vi "Test Asic Rate Scan original con offset analogico.vi"(8 "Error IN":errorcluster, 11 "Config Test IN":T2={"Config HW"={"VISA Rigol DP832"="Rigol_DP832", "Config Rigol DP832"=[{"Channel"=0, "V Limit"=5.5, "I Limit"=0.5, "V Out"=5.0}, {"Channel"=1, "V Limit"=5.5, "I Limit"=0.8, "V Out"=5.0}, {"Channel"=2, "V Limit"=5.5, "I Limit"=0.2, "V Out"=0.0}], "CTA Test#"="CTA013 A", "FT_Handle"=0, "Espera acceso FT"=10}, "Config Test"=[{"Vasic"=2.8, "Global Reset"=FALSE, "Test Register?"=FALSE, "Test ADC?"=FALSE, "Test ADC"={"Repeats ADC"=100, "Max Desviation"=0.1}, "Limits ADC"={"Low"=[1.9, 1.3, 0.65, 0.0, 1.6, 1.4, 1.4, 0.9, 2.1, 0.85, 1.9], "High"=[2.1, 1.5, 0.85, 0.1, 1.4, 1.2, 1.2, 0.7, 1.9, 0.65, 1.7]}, "Test Max PN Min NP?"=FALSE, "Limits Max PN Min NP"={"Max P Upper"=2.177000045776367, "Min P Upper"=1.474, "Max N Upper"=1.475, "Min N Upper"=0.818, "Max P Lower"=1.888, "Min P Lower "=1.321, "Max N Lower"=1.322, "Min N Lower"=0.73}, "Test Rate Scan?"=FALSE, "Vin Rate Scan"=[], "Limits Rate Scan"={"High"=[0.15, 0.242, 0.331, 0.425, 0.512, 0.6, 0.688, 0.774, 0.847, 0.91], "Low"=[0.021, 0.11, 0.189, 0.27, 0.347, 0.421, 0.487, 0.551, 0.601, 0.635]}, "Test Rate Scan Adders?"=FALSE, "Vin Rate Adders"=[], "Limits Rate Scan adders"={"High"=[], "Low"=[]}, "Test offset analog?"=FALSE, "Lim Offset Analog"={"Max Analog"=0.05, "Min Analog"=-0.05}, "Test offset digital?"=FALSE, "Lim offset Dig"={"Max Dig"=0.05}, "Vasic real f.a."=2.8, "IBIAS"=FALSE, "VALUE IBIAS"=63}, {"Vasic"=2.8, "Global Reset"=FALSE, "Test Register?"=FALSE, "Test ADC?"=FALSE, "Test ADC"={"Repeats ADC"=100, "Max Desviation"=0.1}, "Limits ADC"={"Low"=[1.9, 1.3, 0.65, 0.0, 1.6, 1.4, 1.4, 0.9, 2.1, 0.85, 1.9], "High"=[2.1, 1.5, 0.85, 0.1, 1.4, 1.2, 1.2, 0.7, 1.9, 0.65, 1.7]}, "Test Max PN Min NP?"=FALSE, "Limits Max PN Min NP"={"Max P Upper"=2.177000045776367, "Min P Upper"=1.474, "Max N Upper"=1.475, "Min N Upper"=0.818, "Max P Lower"=1.888, "Min P Lower "=1.321, "Max N Lower"=1.322, "Min N Lower"=0.73}, "Test Rate Scan?"=FALSE, "Vin Rate Scan"=[], "Limits Rate Scan"={"High"=[0.15, 0.242, 0.331, 0.425, 0.512, 0.6, 0.688, 0.774, 0.847, 0.91], "Low"=[0.021, 0.11, 0.189, 0.27, 0.347, 0.421, 0.487, 0.551, 0.601, 0.635]}, "Test Rate Scan Adders?"=FALSE, "Vin Rate Adders"=[], "Limits Rate Scan adders"={"High"=[], "Low"=[]}, "Test offset analog?"=FALSE, "Lim Offset Analog"={"Max Analog"=0.05, "Min Analog"=-0.05}, "Test offset digital?"=FALSE, "Lim offset Dig"={"Max Dig"=0.05}, "Vasic real f.a."=2.8, "IBIAS"=FALSE, "VALUE IBIAS"=63}, {"Vasic"=2.8, "Global Reset"=FALSE, "Test Register?"=FALSE, "Test ADC?"=FALSE, "Test ADC"={"Repeats ADC"=100, "Max Desviation"=0.1}, "Limits ADC"={"Low"=[1.9, 1.3, 0.65, 0.0, 1.6, 1.4, 1.4, 0.9, 2.1, 0.85, 1.9], "High"=[2.1, 1.5, 0.85, 0.1, 1.4, 1.2, 1.2, 0.7, 1.9, 0.65, 1.7]}, "Test Max PN Min NP?"=FALSE, "Limits Max PN Min NP"={"Max P Upper"=2.177000045776367, "Min P Upper"=1.474, "Max N Upper"=1.475, "Min N Upper"=0.818, "Max P Lower"=1.888, "Min P Lower "=1.321, "Max N Lower"=1.322, "Min N Lower"=0.73}, "Test Rate Scan?"=FALSE, "Vin Rate Scan"=[], "Limits Rate Scan"={"High"=[0.15, 0.242, 0.331, 0.425, 0.512, 0.6, 0.688, 0.774, 0.847, 0.91], "Low"=[0.021, 0.11, 0.189, 0.27, 0.347, 0.421, 0.487, 0.551, 0.601, 0.635]}, "Test Rate Scan Adders?"=FALSE, "Vin Rate Adders"=[], "Limits Rate Scan adders"={"High"=[], "Low"=[]}, "Test offset analog?"=FALSE, "Lim Offset Analog"={"Max Analog"=0.05, "Min Analog"=-0.05}, "Test offset digital?"=FALSE, "Lim offset Dig"={"Max Dig"=0.05}, "Vasic real f.a."=2.8, "IBIAS"=FALSE, "VALUE IBIAS"=63}, {"Vasic"=2.8, "Global Reset"=FALSE, "Test Register?"=FALSE, "Test ADC?"=FALSE, "Test ADC"={"Repeats ADC"=100, "Max Desviation"=0.1}, "Limits ADC"={"Low"=[1.9, 1.3, 0.65, 0.0, 1.6, 1.4, 1.4, 0.9, 2.1, 0.85, 1.9], "High"=[2.1, 1.5, 0.85, 0.1, 1.4, 1.2, 1.2, 0.7, 1.9, 0.65, 1.7]}, "Test Max PN Min NP?"=FALSE, "Limits Max PN Min NP"={"Max P Upper"=2.177000045776367, "Min P Upper"=1.474, "Max N Upper"=1.475, "Min N Upper"=0.818, "Max P Lower"=1.888, "Min P Lower "=1.321, "Max N Lower"=1.322, "Min N Lower"=0.73}, "Test Rate Scan?"=FALSE, "Vin Rate Scan"=[], "Limits Rate Scan"={"High"=[0.15, 0.242, 0.331, 0.425, 0.512, 0.6, 0.688, 0.774, 0.847, 0.91], "Low"=[0.021, 0.11, 0.189, 0.27, 0.347, 0.421, 0.487, 0.551, 0.601, 0.635]}, "Test Rate Scan Adders?"=FALSE, "Vin Rate Adders"=[], "Limits Rate Scan adders"={"High"=[], "Low"=[]}, "Test offset analog?"=FALSE, "Lim Offset Analog"={"Max Analog"=0.05, "Min Analog"=-0.05}, "Test offset digital?"=FALSE, "Lim offset Dig"={"Max Dig"=0.05}, "Vasic real f.a."=2.8, "IBIAS"=FALSE, "VALUE IBIAS"=63}], "Result"=[], "Execucion Test"={"Vasic Actual"=0}, "Config VGA"={"Theoretical Voltage"=[], "Real Voltage"=[102.85, 207.14, 299.57, 404.85, 495.71, 606.85, 697.71, 801.14, 897.14, 998.85], "Pulse Width"=57344, "Frecuency Pulse"=1000000.0, "VGA Gain"=[9, 16, 24, 34, 43, 52, 61, 72, 81, 93]}, "Test Info"={"Asic"="", "Operator"="", "Place"="", "Time start"=timestamp(0 s since 1904-01-01), "Time stop"=timestamp(0 s since 1904-01-01)}, "Info machine"={"SO"="", "SO Name"="", "SO Ver"="", "SO Build"="", "CPU"="", "APP"="", "APP YEAR"="", "APP ver"="", "APP User"="", "APP Serail"="", "MAC"=[], "PC NAME"=[], "PC IP"=[], "BIOS MANU"="", "BIOS NAME"="", "BIOS SERIAL"="", "BOARD MANU"="", "BOARD NAME"="", "BOARD SERIAL"="", "Driver Version"="", "Library Version"="", "FPGA Ver"=0, "ID CTA board"=0, "LAST BOOT"="", "LABVIEW Ver"=0}} {"Config VGA"."Theoretical Voltage" format="%1.4f"; "Config VGA"."VGA Gain" format="%02x"; "Config VGA"."Frecuency Pulse" format="%0_2p"; "Config VGA"."Pulse Width" format="%04x"; "Config VGA"."Real Voltage" format="%1.5f"; "Config Test"."VALUE IBIAS" max=63 step=1; "Config Test"."Vasic real f.a." min=2.8 max=3.8 step=0.01 format="%.2g"; "Config Test"."Limits Rate Scan adders"."Low" format="%1.3f"; "Config Test"."Limits Rate Scan adders"."High" format="%1.3f"; "Config Test"."Limits ADC"."High" format="%1.4f"; "Config Test"."Limits ADC"."Low" format="%1.3f"; "Config Test"."Lim offset Dig"."Max Dig" format="%.3g"; "Config Test"."Lim Offset Analog"."Min Analog" format="%.3g"; "Config Test"."Lim Offset Analog"."Max Analog" format="%.3g"; "Config Test"."Limits Rate Scan"."Low" format="%1.4f"; "Config Test"."Limits Rate Scan"."High" format="%1.3f"; "Config Test"."Limits Max PN Min NP"."Min P Upper" format="%.3g"; "Config Test"."Limits Max PN Min NP"."Min P Lower" format="%.3g"; "Config Test"."Limits Max PN Min NP"."Max N Lower" format="%.3g"; "Config Test"."Limits Max PN Min NP"."Max N Upper" format="%.3g"; "Config Test"."Limits Max PN Min NP"."Min N Lower" format="%.3g"; "Config Test"."Limits Max PN Min NP"."Min N Upper" format="%.3g"; "Config Test"."Limits Max PN Min NP"."Max P Upper" format="%.3g"; "Config Test"."Limits Max PN Min NP"."Max P Lower" format="%.3g"; "Config Test"."Vasic" min=2.8 max=3.8 step=0.01 format="%.2g"; "Config HW"."Config Rigol DP832"."Channel" items=["+30V Channel 1", "+30V Channel 2", "+5V Channel 3"]; "Config HW"."Config Rigol DP832"."V Limit" format="%.1g"; "Config HW"."Config Rigol DP832"."I Limit" format="%.1g"; "Config HW"."Config Rigol DP832"."V Out" format="%.1g"; "Result"."Test Registros"."Read W/R" format="%04x"; "Result"."Test Registros"."Pattern W/R" format="%04x"; "Result"."Test Registros"."Read Default" format="%04x"; "Result"."Test Registros"."Pattern Default" format="%04x"}) -> (0 "Error OUT":errorcluster, 2 "Rate scan all ok":bool, 3 "Config Test OUT":T2={"Config HW"={"VISA Rigol DP832"="Rigol_DP832", "Config Rigol DP832"=[{"Channel"=0, "V Limit"=5.5, "I Limit"=0.5, "V Out"=5.0}, {"Channel"=1, "V Limit"=5.5, "I Limit"=0.8, "V Out"=5.0}, {"Channel"=2, "V Limit"=5.5, "I Limit"=0.2, "V Out"=0.0}], "CTA Test#"="CTA013 A", "FT_Handle"=0, "Espera acceso FT"=10}, "Config Test"=[{"Vasic"=2.8, "Global Reset"=FALSE, "Test Register?"=FALSE, "Test ADC?"=FALSE, "Test ADC"={"Repeats ADC"=100, "Max Desviation"=0.1}, "Limits ADC"={"Low"=[1.9, 1.3, 0.65, 0.0, 1.6, 1.4, 1.4, 0.9, 2.1, 0.85, 1.9], "High"=[2.1, 1.5, 0.85, 0.1, 1.4, 1.2, 1.2, 0.7, 1.9, 0.65, 1.7]}, "Test Max PN Min NP?"=FALSE, "Limits Max PN Min NP"={"Max P Upper"=2.177000045776367, "Min P Upper"=1.474, "Max N Upper"=1.475, "Min N Upper"=0.818, "Max P Lower"=1.888, "Min P Lower "=1.321, "Max N Lower"=1.322, "Min N Lower"=0.73}, "Test Rate Scan?"=FALSE, "Vin Rate Scan"=[], "Limits Rate Scan"={"High"=[0.15, 0.242, 0.331, 0.425, 0.512, 0.6, 0.688, 0.774, 0.847, 0.91], "Low"=[0.021, 0.11, 0.189, 0.27, 0.347, 0.421, 0.487, 0.551, 0.601, 0.635]}, "Test Rate Scan Adders?"=FALSE, "Vin Rate Adders"=[], "Limits Rate Scan adders"={"High"=[], "Low"=[]}, "Test offset analog?"=FALSE, "Lim Offset Analog"={"Max Analog"=0.05, "Min Analog"=-0.05}, "Test offset digital?"=FALSE, "Lim offset Dig"={"Max Dig"=0.05}, "Vasic real f.a."=2.8, "IBIAS"=FALSE, "VALUE IBIAS"=63}, {"Vasic"=2.8, "Global Reset"=FALSE, "Test Register?"=FALSE, "Test ADC?"=FALSE, "Test ADC"={"Repeats ADC"=100, "Max Desviation"=0.1}, "Limits ADC"={"Low"=[1.9, 1.3, 0.65, 0.0, 1.6, 1.4, 1.4, 0.9, 2.1, 0.85, 1.9], "High"=[2.1, 1.5, 0.85, 0.1, 1.4, 1.2, 1.2, 0.7, 1.9, 0.65, 1.7]}, "Test Max PN Min NP?"=FALSE, "Limits Max PN Min NP"={"Max P Upper"=2.177000045776367, "Min P Upper"=1.474, "Max N Upper"=1.475, "Min N Upper"=0.818, "Max P Lower"=1.888, "Min P Lower "=1.321, "Max N Lower"=1.322, "Min N Lower"=0.73}, "Test Rate Scan?"=FALSE, "Vin Rate Scan"=[], "Limits Rate Scan"={"High"=[0.15, 0.242, 0.331, 0.425, 0.512, 0.6, 0.688, 0.774, 0.847, 0.91], "Low"=[0.021, 0.11, 0.189, 0.27, 0.347, 0.421, 0.487, 0.551, 0.601, 0.635]}, "Test Rate Scan Adders?"=FALSE, "Vin Rate Adders"=[], "Limits Rate Scan adders"={"High"=[], "Low"=[]}, "Test offset analog?"=FALSE, "Lim Offset Analog"={"Max Analog"=0.05, "Min Analog"=-0.05}, "Test offset digital?"=FALSE, "Lim offset Dig"={"Max Dig"=0.05}, "Vasic real f.a."=2.8, "IBIAS"=FALSE, "VALUE IBIAS"=63}, {"Vasic"=2.8, "Global Reset"=FALSE, "Test Register?"=FALSE, "Test ADC?"=FALSE, "Test ADC"={"Repeats ADC"=100, "Max Desviation"=0.1}, "Limits ADC"={"Low"=[1.9, 1.3, 0.65, 0.0, 1.6, 1.4, 1.4, 0.9, 2.1, 0.85, 1.9], "High"=[2.1, 1.5, 0.85, 0.1, 1.4, 1.2, 1.2, 0.7, 1.9, 0.65, 1.7]}, "Test Max PN Min NP?"=FALSE, "Limits Max PN Min NP"={"Max P Upper"=2.177000045776367, "Min P Upper"=1.474, "Max N Upper"=1.475, "Min N Upper"=0.818, "Max P Lower"=1.888, "Min P Lower "=1.321, "Max N Lower"=1.322, "Min N Lower"=0.73}, "Test Rate Scan?"=FALSE, "Vin Rate Scan"=[], "Limits Rate Scan"={"High"=[0.15, 0.242, 0.331, 0.425, 0.512, 0.6, 0.688, 0.774, 0.847, 0.91], "Low"=[0.021, 0.11, 0.189, 0.27, 0.347, 0.421, 0.487, 0.551, 0.601, 0.635]}, "Test Rate Scan Adders?"=FALSE, "Vin Rate Adders"=[], "Limits Rate Scan adders"={"High"=[], "Low"=[]}, "Test offset analog?"=FALSE, "Lim Offset Analog"={"Max Analog"=0.05, "Min Analog"=-0.05}, "Test offset digital?"=FALSE, "Lim offset Dig"={"Max Dig"=0.05}, "Vasic real f.a."=2.8, "IBIAS"=FALSE, "VALUE IBIAS"=63}, {"Vasic"=2.8, "Global Reset"=FALSE, "Test Register?"=FALSE, "Test ADC?"=FALSE, "Test ADC"={"Repeats ADC"=100, "Max Desviation"=0.1}, "Limits ADC"={"Low"=[1.9, 1.3, 0.65, 0.0, 1.6, 1.4, 1.4, 0.9, 2.1, 0.85, 1.9], "High"=[2.1, 1.5, 0.85, 0.1, 1.4, 1.2, 1.2, 0.7, 1.9, 0.65, 1.7]}, "Test Max PN Min NP?"=FALSE, "Limits Max PN Min NP"={"Max P Upper"=2.177000045776367, "Min P Upper"=1.474, "Max N Upper"=1.475, "Min N Upper"=0.818, "Max P Lower"=1.888, "Min P Lower "=1.321, "Max N Lower"=1.322, "Min N Lower"=0.73}, "Test Rate Scan?"=FALSE, "Vin Rate Scan"=[], "Limits Rate Scan"={"High"=[0.15, 0.242, 0.331, 0.425, 0.512, 0.6, 0.688, 0.774, 0.847, 0.91], "Low"=[0.021, 0.11, 0.189, 0.27, 0.347, 0.421, 0.487, 0.551, 0.601, 0.635]}, "Test Rate Scan Adders?"=FALSE, "Vin Rate Adders"=[], "Limits Rate Scan adders"={"High"=[], "Low"=[]}, "Test offset analog?"=FALSE, "Lim Offset Analog"={"Max Analog"=0.05, "Min Analog"=-0.05}, "Test offset digital?"=FALSE, "Lim offset Dig"={"Max Dig"=0.05}, "Vasic real f.a."=2.8, "IBIAS"=FALSE, "VALUE IBIAS"=63}], "Result"=[], "Execucion Test"={"Vasic Actual"=0}, "Config VGA"={"Theoretical Voltage"=[], "Real Voltage"=[102.85, 207.14, 299.57, 404.85, 495.71, 606.85, 697.71, 801.14, 897.14, 998.85], "Pulse Width"=57344, "Frecuency Pulse"=1000000.0, "VGA Gain"=[9, 16, 24, 34, 43, 52, 61, 72, 81, 93]}, "Test Info"={"Asic"="", "Operator"="", "Place"="", "Time start"=timestamp(0 s since 1904-01-01), "Time stop"=timestamp(0 s since 1904-01-01)}, "Info machine"={"SO"="", "SO Name"="", "SO Ver"="", "SO Build"="", "CPU"="", "APP"="", "APP YEAR"="", "APP ver"="", "APP User"="", "APP Serail"="", "MAC"=[], "PC NAME"=[], "PC IP"=[], "BIOS MANU"="", "BIOS NAME"="", "BIOS SERIAL"="", "BOARD MANU"="", "BOARD NAME"="", "BOARD SERIAL"="", "Driver Version"="", "Library Version"="", "FPGA Ver"=0, "ID CTA board"=0, "LAST BOOT"="", "LABVIEW Ver"=0}} {"Config VGA"."Theoretical Voltage" format="%1.4f"; "Config VGA"."VGA Gain" format="%02x"; "Config VGA"."Frecuency Pulse" format="%0_2p"; "Config VGA"."Pulse Width" format="%04x"; "Config VGA"."Real Voltage" format="%1.5f"; "Config Test"."VALUE IBIAS" max=63 step=1; "Config Test"."Vasic real f.a." min=2.8 max=3.8 step=0.01 format="%.2g"; "Config Test"."Limits Rate Scan adders"."Low" format="%1.3f"; "Config Test"."Limits Rate Scan adders"."High" format="%1.3f"; "Config Test"."Limits ADC"."High" format="%1.4f"; "Config Test"."Limits ADC"."Low" format="%1.3f"; "Config Test"."Lim offset Dig"."Max Dig" format="%.3g"; "Config Test"."Lim Offset Analog"."Min Analog" format="%.3g"; "Config Test"."Lim Offset Analog"."Max Analog" format="%.3g"; "Config Test"."Limits Rate Scan"."Low" format="%1.4f"; "Config Test"."Limits Rate Scan"."High" format="%1.3f"; "Config Test"."Limits Max PN Min NP"."Min P Upper" format="%.3g"; "Config Test"."Limits Max PN Min NP"."Min P Lower" format="%.3g"; "Config Test"."Limits Max PN Min NP"."Max N Lower" format="%.3g"; "Config Test"."Limits Max PN Min NP"."Max N Upper" format="%.3g"; "Config Test"."Limits Max PN Min NP"."Min N Lower" format="%.3g"; "Config Test"."Limits Max PN Min NP"."Min N Upper" format="%.3g"; "Config Test"."Limits Max PN Min NP"."Max P Upper" format="%.3g"; "Config Test"."Limits Max PN Min NP"."Max P Lower" format="%.3g"; "Config Test"."Vasic" min=2.8 max=3.8 step=0.01 format="%.2g"; "Config HW"."Config Rigol DP832"."Channel" items=["+30V Channel 1", "+30V Channel 2", "+5V Channel 3"]; "Config HW"."Config Rigol DP832"."V Limit" format="%.1g"; "Config HW"."Config Rigol DP832"."I Limit" format="%.1g"; "Config HW"."Config Rigol DP832"."V Out" format="%.1g"; "Result"."Test Registros"."Read W/R" format="%04x"; "Result"."Test Registros"."Pattern W/R" format="%04x"; "Result"."Test Registros"."Read Default" format="%04x"; "Result"."Test Registros"."Pattern Default" format="%04x"})   [LabVIEW 2009]
uses:
  Test.ctl
  TEST.TEST CONFIG HW.ctl
  Rigol DP832/DP832_Control Channels.ctl
  TEST.TEST CONFIG TEST MATRIZ.ctl
  TEST.TEST CONFIG TEST.ctl
  TEST.TEST RESULT.ctl
  test_result fvasic.ctl
  TEST.TEST EXECUTION TEST.ctl
  TEST.TEST CONFIG VGA.ctl
  TEST.TEST TEST INFO.ctl
  TEST.TEST INFO PC.ctl
  Global.Salir Ya.vi
panel:
  out "subarray":dbl[][](array[numeric])
  in  "DAC\nTH0,TH1,TH2":u16
  in  "Tab Control":enum32{"Page 1", "Page 2"}(tab)
  out "%":u8 format="%02d%%"
  out "B":u8(slide) scale=0.0..100.0
  out "Indicador":string
  out "Comparation LLTH":bool[][][](array[boolean])
  out "Comparation HLTH":bool[][][](array[boolean])
  out "Reference":T1
  out "DAC TH3,TH4,TH5":u16
  out "LLTHx":dbl
  out "DAC TH0,TH1,TH2":u16
  out "HLTHx":dbl
  out "Volt LLTH (salida B)":dbl[][][](array[numeric])
  out "Volt HLTH (salida A)":dbl[][][](array[numeric])
  out "DAC TH3,TH4,TH5":u16[][][](array[numeric])
  out "DAC TH0,TH1,TH2":u16[][][](array[numeric])
  # "Vin Asic"
  # "Canal"
  # "Sumador"
  # "Test ASIC. Rate Scan"
  # "Modo 2\nModo 3\nModo 4\nModo 2\nModo 3\nModo 4"
  # "Modo 2\nModo 3\nModo 4\nModo 2\nModo 3\nModo 4"
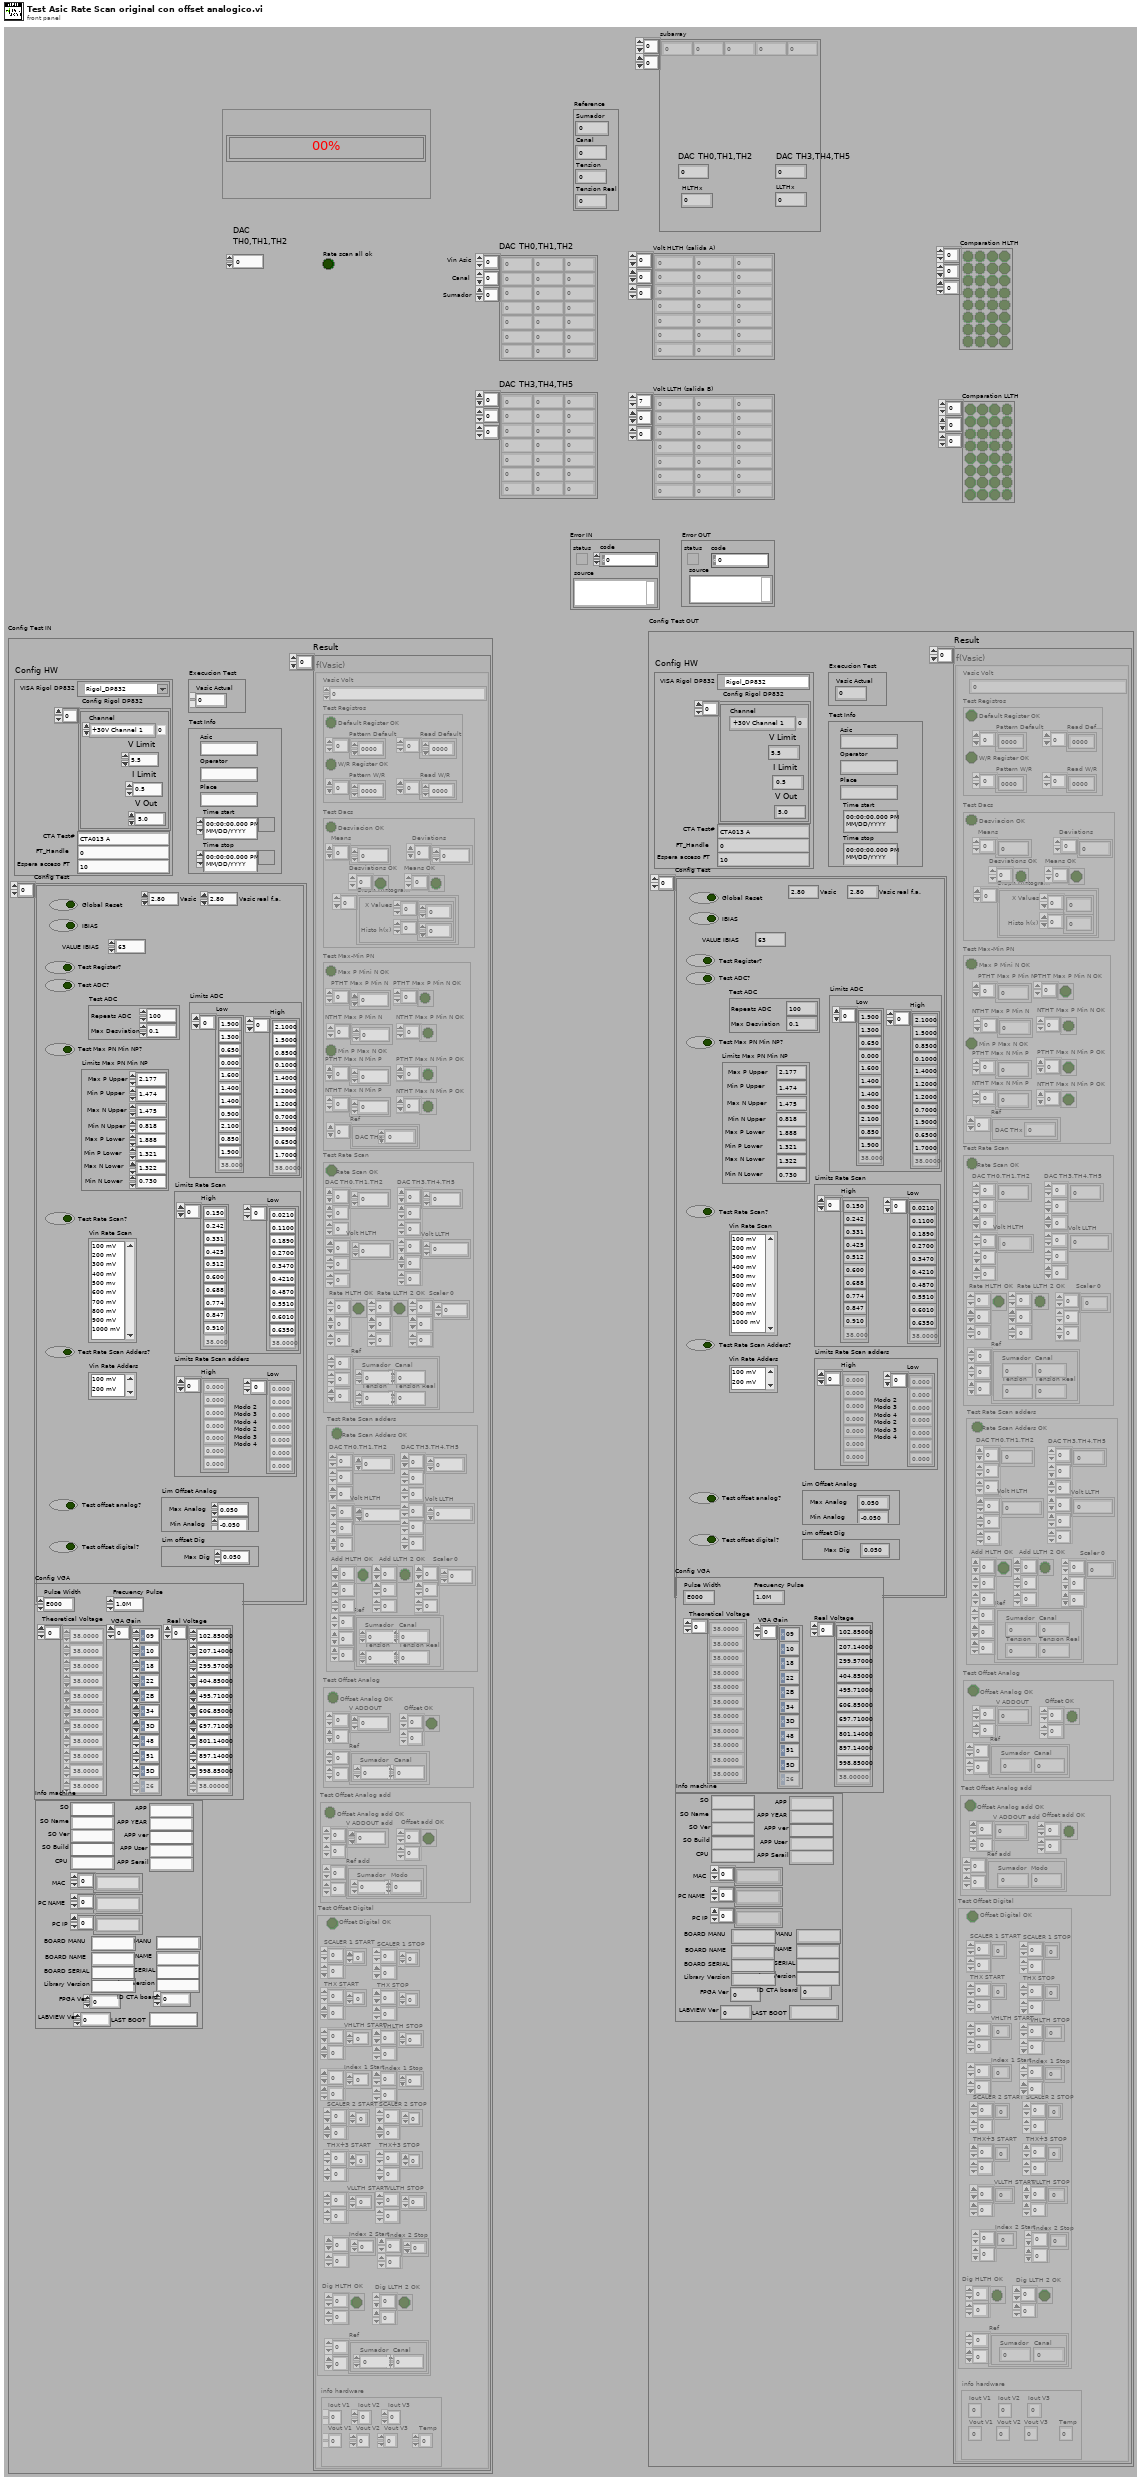
[diagram p1: front panel]
types:
  T1 = cluster{"Sumador":u8, "Canal":u8, "Tension":u8, "Tension Real":dbl}
  T2 = typedef "Test.ctl" = cluster{"Config HW":T3, "Config Test":T5, "Result":T7, "Execucion Test":T9, "Config VGA":T10, "Test Info":T11, "Info machine":T12}
  T3 = typedef "TEST.TEST CONFIG HW.ctl" = cluster{"VISA Rigol DP832":refnum<visa-resource-name>, "Config Rigol DP832":cluster{"Channel":T4, "V Limit":dbl, "I Limit":dbl, "V Out":dbl}[], "CTA Test#":string, "FT_Handle":u32, "Espera acceso FT":u32}
  T4 = typedef "DP832_Control Channels.ctl" = i32
  T5 = typedef "TEST.TEST CONFIG TEST MATRIZ.ctl" = T6[]
  T6 = typedef "TEST.TEST CONFIG TEST.ctl" = cluster{"Vasic":dbl, "Global Reset":bool, "Test Register?":bool, "Test ADC?":bool, "Test ADC":cluster{"Repeats ADC":i32, "Max Desviation":dbl}, "Limits ADC":cluster{"Low":dbl[], "High":dbl[]}, "Test Max PN Min NP?":bool, "Limits Max PN Min NP":cluster{"Max P Upper":dbl, "Min P Upper":dbl, "Max N Upper":dbl, "Min N Upper":dbl, "Max P Lower":dbl, "Min P Lower ":dbl, "Max N Lower":dbl, "Min N Lower":dbl}, "Test Rate Scan?":bool, "Vin Rate Scan":i32[], "Limits Rate Scan":cluster{"High":dbl[], "Low":dbl[]}, "Test Rate Scan Adders?":bool, "Vin Rate Adders":i32[], "Limits Rate Scan adders":cluster{"High":dbl[], "Low":dbl[]}, "Test offset analog?":bool, "Lim Offset Analog":cluster{"Max Analog":dbl, "Min Analog":dbl}, "Test offset digital?":bool, "Lim offset Dig":cluster{"Max Dig":dbl}, "Vasic real f.a.":dbl, "IBIAS":bool, "VALUE IBIAS":u8}
  T7 = typedef "TEST.TEST RESULT.ctl" = T8[]
  T8 = typedef "test_result fvasic.ctl" = cluster{"Vasic Volt":i32, "Test Registros":cluster{"Default Register OK":bool, "Pattern Default":u16[], "Read Default":u16[], "W/R Register OK":bool, "Pattern W/R":u16[], "Read W/R":u16[]}, "Test Dacs":cluster{"Desviacion OK":bool, "Means":dbl[], "Deviations":dbl[], "Desviations OK":bool[], "Means OK":bool[], "Graph Histogram":cluster{"X Values":dbl[], "Histo h(x)":i32[]}[]}, "Test Max-Min PN":cluster{"Max P Mini N OK":bool, "PTHT Max P Min N":dbl[], "PTHT Max P Min N OK":bool[], "NTHT Max P Min N":dbl[], "NTHT Max P Min N OK":bool[], "Min P Max N OK":bool, "PTHT Max N Min P":dbl[], "PTHT Max N Min P OK":bool[], "NTHT Max N Min P":dbl[], "NTHT Max N Min P OK":bool[], "Ref":cluster{"DAC THx":u8}[]}, "Test Rate Scan":cluster{"Rate Scan OK":bool, "DAC TH0,TH1,TH2":u16[][][], "Volt HLTH":dbl[][][], "Rate HLTH OK":bool[][][], "DAC TH3,TH4,TH5":u16[][][], "Volt LLTH":dbl[][][], "Rate LLTH 2 OK":bool[][][], "Scaler 0":u16[][][], "Ref":cluster{"Sumador":u8, "Canal":u8, "Tension":u8, "Tension Real":dbl}[][][]}, "Test Rate Scan adders":cluster{"Rate Scan Adders OK":bool, "DAC TH0,TH1,TH2":u16[][][], "Volt HLTH":dbl[][][], "Add HLTH OK":bool[][][], "DAC TH3,TH4,TH5":u16[][][], "Volt LLTH":dbl[][][], "Add LLTH 2 OK":bool[][][], "Scaler 0":u16[][][], "Ref":cluster{"Sumador":u8, "Canal":u8, "Tension":u8, "Tension Real":dbl}[][][]}, "Test Offset Analog":cluster{"Offset Analog OK":bool, "V ADDOUT":dbl[][], "Offset OK":bool[][], "Ref":cluster{"Sumador":u8, "Canal":u8}[][]}, "Test Offset Digital":cluster{"Offset Digital OK":bool, "SCALER 1 START":u16[][], "SCALER 1 STOP":u16[][], "THX START":u16[][], "THX STOP":u16[][], "VHLTH START":dbl[][], "VHLTH STOP":dbl[][], "Index 1 Start":i32[][], "index 1 Stop":i32[][], "SCALER 2 START":u16[][], "SCALER 2 STOP":u16[][], "THX+3 START":u16[][], "THX+3 STOP":u16[][], "VLLTH START":dbl[][], "VLLTH STOP":dbl[][], "Index 2 Start":i32[][], "index 2 Stop":i32[][], "Dig HLTH OK":bool[][], "Dig LLTH 2 OK":bool[][], "Ref":cluster{"Sumador":u8, "Canal":u8}[][]}, "info hardware":cluster{"Iout V1":dbl, "Iout V2":dbl, "Iout V3":dbl, "Vout V1":dbl, "Vout V2":dbl, "Vout V3":dbl, "Temp":dbl}, "Test Offset Analog add":cluster{"Offset Analog add OK":bool, "V ADDOUT add":dbl[][], "Offset add OK":bool[][], "Ref add":cluster{"Sumador":u8, "Modo":u8}[][]}}
  T9 = typedef "TEST.TEST EXECUTION TEST.ctl" = cluster{"Vasic Actual":i32}
  T10 = typedef "TEST.TEST CONFIG VGA.ctl" = cluster{"Theoretical Voltage":dbl[], "Real Voltage":dbl[], "Pulse Width":u16, "Frecuency Pulse":dbl, "VGA Gain":u8[]}
  T11 = typedef "TEST.TEST TEST INFO.ctl" = cluster{"Asic":string, "Operator":string, "Place":string, "Time start":timestamp, "Time stop":timestamp}
  T12 = typedef "TEST.TEST INFO PC.ctl" = cluster{"SO":string, "SO Name":string, "SO Ver":string, "SO Build":string, "CPU":string, "APP":string, "APP YEAR":string, "APP ver":string, "APP User":string, "APP Serail":string, "MAC":string[], "PC NAME":string[], "PC IP":string[], "BIOS MANU":string, "BIOS NAME":string, "BIOS SERIAL":string, "BOARD MANU":string, "BOARD NAME":string, "BOARD SERIAL":string, "Driver Version":string, "Library Version":string, "FPGA Ver":u8, "ID CTA board":u64, "LAST BOOT":string, "LABVIEW Ver":u32}
  T13 = enum16{"Always On", "Always Off", "Off While Running"}
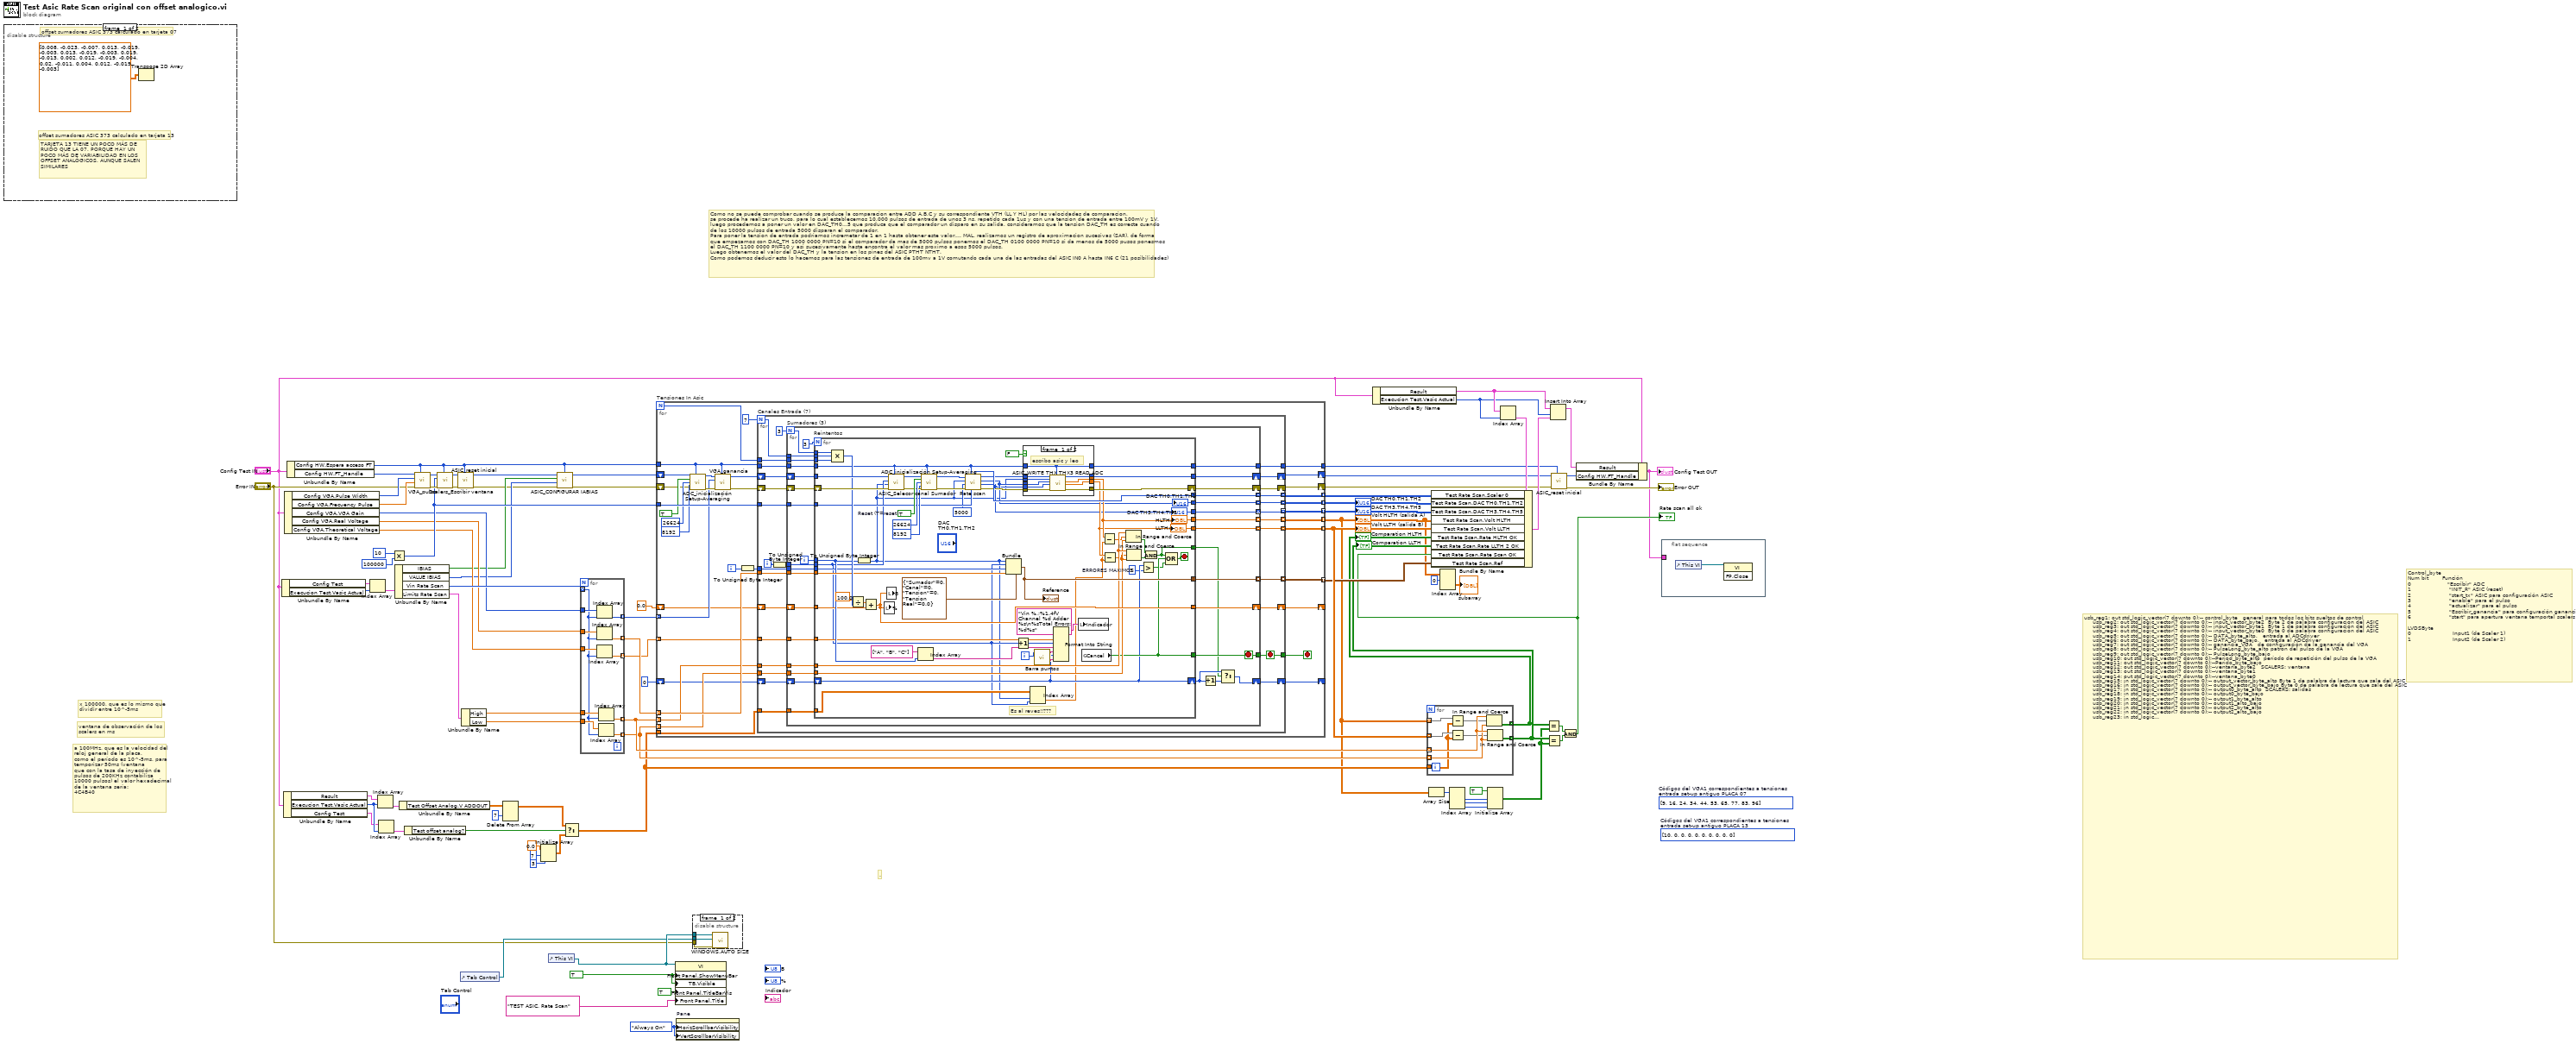
[diagram p0: block diagram]
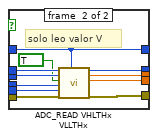
[diagram p4: hidden frame]
diagram:
  w1 = T13."Always On" ("Horizontal Scrollbar Visibility")
  w41 = TRUE ("Front Panel Window:Show Menu Bar")
  (unwired) u8[] [10, 0, 0, 0, 0, 0, 0, 0, 0, 0]  # Códigos del VGA1 correspondientes a tensiones entrada set-up antiguo PLACA 13
  (unwired) u8[] [9, 16, 24, 34, 44, 53, 65, 77, 83, 96]  # Códigos del VGA1 correspondientes a tensiones entrada set-up antiguo PLACA 07
  # "."
  # "Como no se puede comprobar cuando se produce la comparacion entre ADD A,B,C y su correspondiente VTH (LL Y HL) por las velocidades de comparacion,\nse procede ha realizar un truco, para lo cual establecemos 10.000 pulsos de entrada de unos 3 ns, repetido cada 1us y con una tension de entrada entre 100mV y 1V,\nluego procedemos a poner un valor en DAC_TH0...5 que produca que el comparador un disparo en su salida, consideramos que la tension DAC_TH es correcta cuando\nde los 10000 pulsos de entrada 5000 disparan el comparador.\nPara poner la tension de entrada podriamos incremetar de 1 en 1 hasta obtener este valor.... MAL. realizamos un registro de aproximacion sucesivas (SAR), de forma\nque empezamos con DAC_TH 1000 0000 PN=10 si el comparador da mas de 5000 pulsos ponemos el DAC_TH 0100 0000 PN=10 si da menos de 5000 pusos ponesmos\nel DAC_TH 1100 0000 PN=10 y asi sucesivamente hasta encontra el valor mas proximo a esos 5000 pulsos. \nLuego obtenemos el valor del DAC_TH y la tension en los pines del ASIC PTHT NTHT.\nComo podemos deducir esto lo hacemos para las tensiones de entrada de 100mv a 1V comutando cada una de las entradas del ASIC IN0 A hasta IN6 C (21 posibilidades)"
  # "Control_byte\nNum bit        Función\n0                     \"Escribir\" ADC\n1                      \"INIT_R\" ASIC (reset)\n2                      \"start_tx\" ASIC para configuración ASIC\n3                      \"enable\" para el pulso\n4                      \"actualizar\" para el pulso\n5                      \"Escribir_ganancia\" para configuración ganancia\n6                      \"start\" para apertura ventana temportal scalers\n\nLVDSByte\n0                        Input1 (de Scaler 1)\n1                        Input2 (de Scaler 2)"
  # "usb_reg1: out std_logic_vector(7 downto 0);-- control_byte\t\t\tgeneral para todos los bits sueltos de control\n\t\t\t  usb_reg2: out std_logic_vector(7 downto 0);-- input_vector_byte2 \tByte 2 de palabra configuración del ASIC\n\t\t\t  usb_reg3: out std_logic_vector(7 downto 0);-- input_vector_byte1 \tByte 1 de palabra configuración del ASIC\n\t\t\t  usb_reg4: out std_logic_vector(7 downto 0);-- input_vector_byte0 \tByte 0 de palabra configuración del ASIC\n\t\t\t  usb_reg5: out std_logic_vector(7 downto 0);-- DATA_byte_alto, \t\tentrada al ADCdriver\n\t\t\t  usb_reg6: out std_logic_vector(7 downto 0);-- DATA_byte_bajo, \t\tentrada al ADCdriver\n\t\t\t  usb_reg7: out std_logic_vector(7 downto 0);-- ganancia_VGA\t\t\tde configuración de la ganancia del VGA\n\t\t\t  usb_reg8: out std_logic_vector(7 downto 0);-- PulseLong_byte_alto\tpatrón del pulso de la VGA\n\t\t\t  usb_reg9: out std_logic_vector(7 downto 0);-- PulseLong_byte_bajo\n\t\t\t  usb_reg10: out std_logic_vector(7 downto 0);--Period_byte_alto\t\tperíodo de repetición del pulso de la VGA\n\t\t\t  usb_reg11: out std_logic_vector(7 downto 0);--Perido_byte_bajo\n\t\t\t  usb_reg12: out std_logic_vector(7 downto 0);--ventana_byte2\t\t\tSCALERS: ventana\n\t\t\t  usb_reg13: out std_logic_vector(7 downto 0);--ventana_byte1\t\n\t\t\t  usb_reg14: out std_logic_vector(7 downto 0);--ventana_byte0\n\t\t\t  usb_reg15: in std_logic_vector(7 downto 0);-- output_vector_byte_alto\tByte 1 de palabra de lectura que sale del ASIC\n\t\t\t  usb_reg16: in std_logic_vector(7 downto 0);-- output_vector_byte_bajo\tByte 0 de palabra de lectura que sale del ASIC\n\t\t\t  usb_reg17: in std_logic_vector(7 downto 0);-- output0_byte_alto\t\tSCALERS: salidas\n\t\t\t  usb_reg18: in std_logic_vector(7 downto 0);-- output0_byte_bajo\n\t\t\t  usb_reg19: in std_logic_vector(7 downto 0);-- output1_byte_alto\n\t\t\t  usb_reg20: in std_logic_vector(7 downto 0);-- output1_alto_bajo \n\t\t\t  usb_reg21: in std_logic_vector(7 downto 0);-- output2_byte_alto \n\t\t\t  usb_reg22: in std_logic_vector(7 downto 0);-- output2_alto_bajo \n\t\t\t  usb_reg23: in std_logic_vector(7 downto 0);-- para el canal_0 del ADCdriver\n\t\t\t  usb_reg24: in std_logic_vector(7 downto 0);\n\t\t\t  usb_reg25: in std_logic_vector(7 downto 0);-- para el canal_1 del ADCdriver\n\t\t\t  usb_reg26: in std_logic_vector(7 downto 0);\n\t\t\t  usb_reg27: in std_logic_vector(7 downto 0);-- para el canal_2 del ADCdriver\n\t\t\t  usb_reg28: in std_logic_vector(7 downto 0);\n\t\t\t  usb_reg29: in std_logic_vector(7 downto 0);-- para el canal_3 del ADCdriver\n\t\t\t  usb_reg30: in std_logic_vector(7 downto 0);\n\t\t\t  usb_reg31: in std_logic_vector(7 downto 0);-- para el canal_4 del ADCdriver\n\t\t\t  usb_reg32: in std_logic_vector(7 downto 0);\n\t\t\t  usb_reg33: in std_logic_vector(7 downto 0);-- para el canal_5 del ADCdriver\n\t\t\t  usb_reg34: in std_logic_vector(7 downto 0);\n\t\t\t  usb_reg35: in std_logic_vector(7 downto 0);-- para el canal_6 del ADCdriver\n\t\t\t  usb_reg36: in std_logic_vector(7 downto 0);\n\t\t\t  usb_reg37: in std_logic_vector(7 downto 0);-- para el canal_7 del ADCdriver\n\t\t\t  usb_reg38: in std_logic_vector(7 downto 0);\n\t\t\t  usb_reg39: in std_logic_vector(7 downto 0);-- para el canal_8 del ADCdriver\n\t\t\t  usb_reg40: in std_logic_vector(7 downto 0);\n\t\t\t  usb_reg41: in std_logic_vector(7 downto 0);-- para el canal_9 del ADCdriver\n\t\t\t  usb_reg42: in std_logic_vector(7 downto 0);\n\t\t\t  usb_reg43: in std_logic_vector(7 downto 0);-- para el canal_10 del ADCdriver\n\t\t\t  usb_reg44: in std_logic_vector(7 downto 0)--;  \n\n     usb_reg55 => LVDSByte"
  # "x 100000, que es lo mismo que dividir entre 10^-5ms"
  # "ventana de observación de los scalers en ms"
  # "a 100MHz, que es la velocidad del reloj general de la placa,\ncomo el período es 10^-5ms, para temporizar 50ms (ventana \nque con la tasa de inyección de pulsos de 200KHz contabiliza \n10000 pulsos) el valor hexadecimal de la ventana sería:\n4C4B40"
  n1 = disable-structure shown="Enabled" {
    frame #0 {
      # "TARJETA 13 TIENE UN POCO MÁS DE \nRUIDO QUE LA 07, PORQUE HAY UN\nPOCO MÁS DE VARIABILIDAD EN LOS \nOFFSET ANALÓGICOS, AUNQUE SALEN\nSIMILARES"
      # "offset sumadores ASIC 373 calculado en tarjeta 13"
      # "offset sumadores ASIC 373 calculado en tarjeta 07"
      n2 = Transpose 2D Array(2D array=dbl[][] [[0.008, -0.023, -0.007], [0.013, -0.019, -0.003], [0.013, -0.019, -0.003], [0.019, -0.013, 0.002], [0.012, -0.019, -0.004], [0.02, -0.011, 0.004], [0.012, -0.019, -0.003]]) -> ()  [unwired: 1 out]
    }
    frame #1 {
    }
  }
  n3 = Unbundle By Name("Config Test IN") -> ("Config Test"=w71:T5, "Execucion Test.Vasic Actual"=w70:i32)
  n4 = Unbundle By Name("Config Test IN") -> ("Result"=w21:T7, "Execucion Test.Vasic Actual"=w17:i32, "Config Test"=w14:T5)
  n5 = Unbundle By Name("Config Test IN") -> ("Config VGA.Pulse Width"=w65:u16, "Config VGA.Frecuency Pulse"=w64:dbl, "Config VGA.VGA Gain"=w63:u8[], "Config VGA.Real Voltage"=w62:dbl[], "Config VGA.Theoretical Voltage"=w34:dbl[])
  n6 = Unbundle By Name("Config Test IN") -> ("Config HW.Espera acceso FT"=w25:u32, "Config HW.FT_Handle"=w79:u32)
  n7 = Index Array(array=w71, index=w70) -> (element=w69:T6)
  n8 = Index Array(array=w21, index=w17) -> (element=w20:T8)
  n9 = Index Array(array=w14, index=w17) -> (element=w16:T6)
  n10 = Multiply(x=u32 10 ("Ventana"), y=u32 100000 ("Ventana")) -> (x*y=w80:u32)
  n11 = Unbundle By Name(w69) -> ("IBIAS"=w27:bool, "VALUE IBIAS"=w26:u8, "Vin Rate Scan"=w68:i32[], "Limits Rate Scan"=w50:cluster{"High":dbl[], "Low":dbl[]})
  n12 = Unbundle By Name(w20) -> ("Test Offset Analog.V ADDOUT"=w18:dbl[][])
  n13 = Unbundle By Name(w16) -> ("Test offset analog?"=w13:bool)
  n14 = call "VGA_pulso.vi"("Espera acceso USB"=w25, "error in"="Error IN", "Frecuencia pulso (0.2 a 1 Mhz)"=w64, "Patrón (E000)"=w65, "ftHandle_in"=w79) -> ("error out"=w83:errorcluster, "ftHandle_out"=w84:u32)  [unwired: 5 in]
  n15 = call "Scalers_Escribir ventana.vi"("Espera acceso USB"=w25, "error in"=w83, "Ventana"=w80, "ftHandle_in"=w84) -> ("error out"=w81:errorcluster, "ftHandle_out"=w82:u32)  [unwired: 6 in]
  n16 = call "ASIC_reset inicial.vi"("Espera acceso USB"=w25, "error in"=w81, "ftHandle_in"=w82) -> ("error out"=w24:errorcluster, "ftHandle_out"=w78:u32)  [unwired: 7 in]
  n17 = control-ref of="Tab Control"() -> (w37:refnum<vi>)
  n18 = Unbundle By Name(w50) -> ("High"=w49:dbl[], "Low"=w48:dbl[])
  n19 = Delete From Array(array=w18, index (row)=7) -> (array with subset deleted=w8:dbl[][])  [unwired: 2 in, 1 out]
  n20 = Initialize Array(0.0, 7 ("dimension size"), 3 ("dimension size")) -> (w9:dbl[][])
  n21 = control-ref of="This VI"() -> (w38:refnum<vi>)
  n22 = call "ASIC_CONFIGURAR IABIAS.vi"("Espera acceso USB"=w25, "error in"=w24, "IBIAS VALUE"=w26, "IBIAS"=w27, "ftHandle_in"=w78) -> ("error out"=w23:errorcluster, "ftHandle_out"=w28:u32)  [unwired: 5 in]
  n23 = Select(t=w8, s=w13, f=w9) -> (s? t:f=w7:dbl[][])
  n24 = for {
    tunnel: w68 -> [w88] mode=indexing
    tunnel: w63 -> [w98]
    tunnel: w62 -> [w91]
    tunnel: [w97] -> w35 mode=indexing
    tunnel: [w96] -> w67 mode=indexing
    tunnel: w49 -> [w95]
    tunnel: w48 -> [w94]
    tunnel: [w93] -> w31 mode=indexing
    tunnel: [w92] -> w30 mode=indexing
    tunnel: w34 -> [w90]
    tunnel: [w89] -> w33 mode=indexing
    n25 = Index Array(array=w91, index=w88) -> (element=w96:dbl)
    n26 = Index Array(array=w90, index=w88) -> (element=w89:dbl)
    n27 = Index Array(array=w98, index=w88) -> (element=w97:u8)
    n28 = Index Array(array=w94, index=w88) -> (element=w92:dbl)
    n29 = Index Array(array=w95, index=w88) -> (element=w93:dbl)
  }
  n30 = for "Tensiones In Asic" {
    N -> [w109]
    shift-right: [w131] -> w43
    shift-left: w28 -> [w122]
    shift-right: [w130] -> w46
    shift-left: w23 -> [w118]
    tunnel: w25 -> [w119]
    tunnel: w80 -> [w133]
    tunnel: [w129] -> w5 mode=indexing
    tunnel: [w128] -> w76 mode=indexing
    tunnel: w35 -> [w120] mode=indexing
    tunnel: [w117] -> w3 mode=indexing
    tunnel: [w116] -> w61 mode=indexing
    tunnel: w67 -> [w114] mode=indexing
    tunnel: [w113] -> w66 mode=indexing
    tunnel: [w111] -> w53 mode=indexing
    tunnel: [w110] -> w42
    tunnel: w33 -> [w108] mode=indexing
    shift-right: [w106] -> _
    shift-left: 0.0 ("x/y") -> [w107]
    tunnel: w31 -> [w104] mode=indexing
    tunnel: w30 -> [w103] mode=indexing
    shift-right: [w101] -> _
    shift-left: u32 0 ("ms wait IN") -> [w102]
    tunnel: w7 -> [w99]
    i -> [w115]
    stop <- w105 stop-if-true
    n31 = call "ADC_inicialización Setup-Averaging.vi"("ftHandle_in 2"=w122, "Espera acceso USB"=w119, "Reset (T=reset)"=TRUE, "Registro Setup (0x6800)"=u16 26624, "Registro Averaging (0x3200)"=u16 8192 ("Registro Setup (0x6800)"), "error in 2"=w118) -> ("ftHandle_out"=w123:u32, "error out"=w124:errorcluster)  [unwired: 8 in]
    n32 = call "VGA_ganancia.vi"("Espera acceso USB"=w119, "error in 2"=w124, "Ganancia"=w120, "ftHandle_in 2"=w123) -> ("error out 2"=w100:errorcluster, "ftHandle_out 2"=w121:u32)  [unwired: 6 in]
    n33 = To Unsigned Byte Integer(number=w115) -> (unsigned 8bit integer=w112:u8)
    n34 = for "Canales Entrada (7)" {
      N: 7 -> [w144]
      tunnel: w119 -> [w158]
      tunnel: w133 -> [w159]
      shift-right: [w155] -> w131
      shift-left: w121 -> [w162]
      shift-right: [w154] -> w130
      shift-left: w100 -> [w161]
      tunnel: [w153] -> w129 mode=indexing
      tunnel: [w152] -> w128 mode=indexing
      tunnel: [w151] -> w117 mode=indexing
      tunnel: [w150] -> w116 mode=indexing
      tunnel: w112 -> [w149]
      tunnel: w114 -> [w148]
      tunnel: [w147] -> w113 mode=indexing
      tunnel: [w146] -> w111 mode=indexing
      tunnel: [w145] -> w110
      tunnel: w109 -> [w143]
      tunnel: w108 -> [w142]
      shift-right: [w140] -> w106
      shift-left: w107 -> [w141]
      tunnel: [w139] -> w105
      tunnel: w104 -> [w138]
      tunnel: w103 -> [w137]
      shift-right: [w135] -> w101
      shift-left: w102 -> [w136]
      tunnel: w99 -> [w134]
      i -> [w160]
      stop <- w139 stop-if-true
      n35 = To Unsigned Byte Integer(number=w160) -> (unsigned 8bit integer=w156:u8)
      n36 = for "Sumadores (3)" {
        N: 3 -> [w184]
        tunnel: w156 -> [w180]
        tunnel: w159 -> [w193]
        tunnel: w158 -> [w186]
        shift-right: [w189] -> w154
        shift-left: w161 -> [w192]
        shift-right: [w190] -> w155
        shift-left: w162 -> [w191]
        tunnel: [w195] -> w153 mode=indexing
        tunnel: [w194] -> w152 mode=indexing
        tunnel: [w173] -> w151 mode=indexing
        tunnel: [w172] -> w150 mode=indexing
        tunnel: w149 -> [w185]
        tunnel: w148 -> [w181]
        tunnel: [w188] -> w147 mode=indexing
        tunnel: [w187] -> w146 mode=indexing
        tunnel: [w164] -> w145
        tunnel: w144 -> [w183]
        tunnel: w143 -> [w182]
        tunnel: w142 -> [w178]
        shift-right: [w176] -> w140
        shift-left: w141 -> [w177]
        tunnel: [w169] -> w139
        tunnel: w138 -> [w175]
        tunnel: w137 -> [w174]
        shift-right: [w168] -> w135
        shift-left: w136 -> [w170]
        tunnel: w134 -> [w163]
        i -> [w179]
        stop <- w169 stop-if-true
        n37 = for "Reintentos" {
          N: 3 -> [_]
          tunnel: [w205] -> w195
          tunnel: [w204] -> w194
          tunnel: w193 -> [w213]
          tunnel: w191 -> [w252]
          tunnel: [w249] -> w190
          tunnel: [w246] -> w188
          tunnel: [w245] -> w187
          tunnel: w186 -> [w212]
          tunnel: w185 -> [w211]
          tunnel: w184 -> [w243]
          tunnel: w183 -> [w242]
          tunnel: w182 -> [w241]
          tunnel: w181 -> [w238]
          tunnel: w180 -> [w197]
          tunnel: w179 -> [w236]
          tunnel: w178 -> [w233]
          tunnel: [w221] -> w169
          tunnel: w175 -> [w227]
          tunnel: w174 -> [w226]
          tunnel: [w225] -> w173
          tunnel: [w224] -> w172
          shift-right: [w248] -> w189
          shift-left: w192 -> [w253]
          tunnel: w177 -> [w230]
          tunnel: [w228] -> w176
          shift-right: [w215] -> w167
          shift-left: w170 -> [w215]
          tunnel: [w218] -> w165
          tunnel: [w203] -> w164
          tunnel: w163 -> [w201]
          i -> [w217]
          stop <- w220 stop-if-true
          w214 = u32 3  # ERRORES MAXIMOS
          w255 = TRUE  # Reset (T=reset)
          # "Es al reves!!???"
          n38 = Compound Arithmetic op=MULTIPLY(w243, w242, w241) -> (w240:i32)
          n39 = Divide(x=100.0, y=w240) -> (x/y=w229:dbl)
          n40 = To Unsigned Byte Integer(number=w236) -> (unsigned 8bit integer=w196:u8)
          n41 = Add(x=w229, y=w230) -> (x+y=w228:dbl)
          n42 = local write "%"(w228) -> ()
          n43 = local write "B"(w228) -> ()
          n44 = call "ASIC_Selecor canal Sumador.vi"("Espera acceso USB"=w212, "error in"=w253, "Sumador"=w196, "Canal"=w197, "ftHandle_in"=w252) -> ("error out"=w251:errorcluster, "ftHandle_out"=w250:u32)  [unwired: 4 in, 1 out]
          n45 = Index Array(array=string[] ["A", "B", "C"], index=w236) -> (element=w235:string)
          n46 = call "ADC_inicialización Setup-Averaging.vi"("ftHandle_in 2"=w250, "Espera acceso USB"=w212, "Reset (T=reset)"=w255, "Registro Setup (0x6800)"=u16 26624, "Registro Averaging (0x3200)"=u16 8192 ("Registro Setup (0x6800)"), "error in 2"=w251) -> ("ftHandle_out"=w210:u32, "error out"=w209:errorcluster)  [unwired: 8 in]
          n47 = call "Rate scan.vi"("T Ventana"=w213, "Espera acceso USB"=w212, "error in 2"=w209, "Valor buscado scalers (5000)"=u16 5000 ("Valor buscado scalers"), "Sumador"=w196, "ftHandle_in 2"=w210) -> ("error out 2"=w207:errorcluster, "DAC\nTH3,TH4,TH5"=w204:u16, "DAC\nTH0,TH1,TH2"=w205:u16, "ftHandle_out 2"=w208:u32, "Scaler 1"=w246:u16)  [unwired: 1 in]
          "DAC TH0,TH1,TH2" <- w205
          "DAC TH3,TH4,TH5" <- w204
          n48 = Bundle(cluster=T1 {"Sumador"=0, "Canal"=0, "Tension"=0, "Tension Real"=0.0}, "Sumador"=w196, "Canal"=w197, "Tension"=w211, "Tension Real"=w238) -> (w245:T1)
          "Reference" <- w245
          n49 = Increment(x=w197) -> (x+1=w232:u8)
          n50 = case shown="False" FALSE {
            tunnel: [w265 w276] -> w249
            tunnel: [w259 w275] -> w248
            tunnel: [w257 w274] -> w225
            tunnel: [w258 w273] -> w224
            tunnel: w212 -> [w256 w266]
            tunnel: w196 -> [w263 w272]
            tunnel: w208 -> [w264 w271]
            tunnel: w207 -> [w260 w270]
            tunnel: w205 -> [w262 w269]
            tunnel: w204 -> [w261 w268]
            tunnel: [w256 w266] -> w203
            frame #0 {
              # "escribo asic y leo"
              n51 = call "ASIC_WRITE THX THX3 READ ADC.vi"("ftHandle_in"=w264, "Sumador"=w263, "THX"=w262, "THX+3"=w261, "error in"=w260, "Espera acceso USB 2"=w256) -> ("ftHandle_out"=w265:u32, "HLTHx"=w257:dbl, "LLTHx"=w258:dbl, "error out"=w259:errorcluster)  [unwired: 10 in]
            }
            frame #1 {
              # "solo leo valor V"
              n52 = call "ADC_READ VHLTHx VLLTHx.vi"("ftHandle_out 2"=w271, "Sumador"=w272, "referenciar"=TRUE, "ref DAC\nTH0,TH1,TH2"=w269, "ref DAC\nTH3,TH4,TH5"=w268, "error out 2"=w270, "Espera acceso FT"=w266) -> ("ftHandle_out"=w276:u32, "HLTHx"=w274:dbl, "LLTHx"=w273:dbl, "error out"=w275:errorcluster)  [unwired: 9 in]
            }
          }
          "HLTHx" <- w225
          "LLTHx" <- w224
          n53 = Index Array(array=w201, index (row)=w196, index (col)=w197) -> (element=w198:dbl)
          n54 = call "Barra puntos.vi"("#N"=w217) -> ("String"=w216:string)  [unwired: 8 in]
          n55 = Format Into String(format string="Vin %,;%1.4fV Channel %d Adder %s\n%sTotal Errors: %d%s", w233, w232, w235, w216, w215, w216) -> (resulting string=w234:string)  [unwired: 2 in, 1 out]
          n56 = local write "Indicador"(w234) -> ()
          n57 = global read "Global.Salir Ya.vi" "Cancel"() -> (w221:bool)
          n58 = Subtract(x=w225, y=w198) -> (x-y=w200:dbl)
          n59 = Subtract(x=w224, y=w198) -> (x-y=w199:dbl)
          n60 = In Range and Coerce(upper limit=w227, x=w200, lower limit=w226) -> (In Range?=w222:bool)  [unwired: 1 out]
          n61 = In Range and Coerce(upper limit=w227, x=w199, lower limit=w226) -> (In Range?=w223:bool)  [unwired: 1 out]
          n62 = Greater?(x=w215, y=w214) -> (0:w219:bool)
          n63 = And(x=w222, y=w223) -> (x .and. y?=w218:bool)
          n64 = Compound Arithmetic op=OR(w218, w221, w219) -> (w220:bool)
        }
        n65 = Increment(x=w167) -> (x+1=w166:u32)
        n66 = Select(t=w167, s=w165, f=w166) -> (s? t:f=w168:u32)
      }
    }
  }
  "DAC TH0,TH1,TH2" <- w5
  "DAC TH3,TH4,TH5" <- w76
  "Volt HLTH (salida A)" <- w3
  "Volt LLTH (salida B)" <- w61
  n67 = property class="VI"(reference=w38, "Front Panel.ShowMenuBar"=w41, "TB.Visible"=w41, "Front Panel.TitleBarVis"=TRUE ("Front Panel Window:Title Bar Visible"), "Front Panel.Title"="TEST ASIC. Rate Scan" ("Front Panel Window:Title")) -> ()  [unwired: 1 in, 2 out]
  n68 = property on="Pane" class="Pane"("HorizScrollbarVisibility"=w1, "VertScrollbarVisibility"=w1) -> ()  [unwired: 2 in, 2 out]
  n69 = disable-structure shown="Enabled" {
    disable-tunnel: w38 -> [w279 _]
    disable-tunnel: w37 -> [w278 _]
    disable-tunnel: "Error IN" -> [w277 _]
    frame #0 {
      n70 = call "WINDOWS.AUTO SIZE.vi"("Error In"=w277, "TAB.AutoAjuste"=w278, "This VI"=w279) -> ()  [unwired: 4 in, 1 out]
    }
    frame #1 {
    }
  }
  n71 = Unbundle By Name("Config Test IN") -> ("Result"=w74:T7, "Execucion Test.Vasic Actual"=w73:i32)
  n72 = for {
    tunnel: w3 -> [w281] mode=indexing
    tunnel: w61 -> [w283] mode=indexing
    tunnel: [w287] -> w6 mode=indexing
    tunnel: [w288] -> w51 mode=indexing
    tunnel: w31 -> [w286] mode=indexing
    tunnel: w30 -> [w285] mode=indexing
    tunnel: w7 -> [w280]
    n73 = Subtract(x=w281, y=w280) -> (x-y=w284:dbl[][])
    n74 = Subtract(x=w283, y=w280) -> (x-y=w282:dbl[][])
    n75 = In Range and Coerce(upper limit=w286, x=w284, lower limit=w285) -> (In Range?=w287:bool[][])  [unwired: 1 out]
    n76 = In Range and Coerce(upper limit=w286, x=w282, lower limit=w285) -> (In Range?=w288:bool[][])  [unwired: 1 out]
  }
  "Comparation HLTH" <- w6
  "Comparation LLTH" <- w51
  n77 = Array Size(array=w3) -> (size(s)=w60:i32[])
  n78 = Index Array(array=w3, index (dim 0)=0 ("index (page)")) -> (element=→"subarray":dbl[][])  [unwired: 2 in]
  n79 = Index Array(array=w60) -> (element #1=w59:i32, element #2=w58:i32, element #3=w57:i32)  [unwired: 3 in]
  n80 = Initialize Array(TRUE, w59, w58, w57) -> (w47:bool[][][])
  n81 = Index Array(array=w74, index=w73) -> (element=w77:T8)
  n82 = Equal?(x=w6, y=w47) -> (x = y?=w55:bool)
  n83 = Equal?(x=w51, y=w47) -> (x = y?=w54:bool)
  n84 = call "ASIC_reset inicial.vi"("Espera acceso USB"=w42, "error in"=w46, "ftHandle_in"=w43) -> ("error out"=→"Error OUT":errorcluster, "ftHandle_out"=w44:u32)  [unwired: 7 in]
  n85 = And(x=w55, y=w54) -> (x .and. y?=w52:bool)
  "Rate scan all ok" <- w52
  n86 = Bundle By Name(cluster=w77, "Test Rate Scan.Scaler 0"=w66, "Test Rate Scan.DAC TH0,TH1,TH2"=w5, "Test Rate Scan.DAC TH3,TH4,TH5"=w76, "Test Rate Scan.Volt HLTH"=w3, "Test Rate Scan.Volt LLTH"=w61, "Test Rate Scan.Rate HLTH OK"=w6, "Test Rate Scan.Rate LLTH 2 OK"=w51, "Test Rate Scan.Rate Scan OK"=w52, "Test Rate Scan.Ref"=w53) -> (w75:T8)
  n87 = Insert Into Array(array=w74, index=w73, new element=w75) -> (w72:T7)
  n88 = Bundle By Name(cluster="Config Test IN", "Result"=w72, "Config HW.FT_Handle"=w44) -> (w15:T2)
  "Config Test OUT" <- w15
  n89 = flat-sequence {
    tunnel: w15 -> [_]
    frame #0 {
      n90 = control-ref of="This VI"() -> (w289:refnum<vi>)
      n91 = invoke class="VI" method="FP.Close"(reference=w289) -> ()  [unwired: 2 in, 3 out]
    }
  }
